vi "Spinner Facade.vi"(0 "Data In":T4, 2 "Display State In":T2, 3 "Container State":T3) -> (6 "Data Out":T4, 7 "Display State Out":T2, 8 "Action":T1)   [LabVIEW 2012, in "Spinner.xctl"]
uses:
  Spinner.xctl
  Spinner Data.ctl
  <vilib>/_xctls/Container State.ctl
  Spinner State.ctl
  <vilib>/_xctls/Action.ctl
  Command.ctl
  <vilib>/_xctls/XControlSupport.lvlib
panel:
  out "Spinner":picture
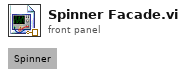
[diagram p1: front panel]
types:
  T1 = typedef "XControlSupport.lvlib/Action.ctl" = cluster{"Data Changed?":bool, "State Changed?":bool, "Action Name":string}
  T2 = typedef "Spinner.xctl/Spinner State.ctl" = cluster{"Min Speed":dbl, "Color":u32, "Max Speed":dbl, "First Run?":bool, "Value":dbl, "Refnum":refnum<vi>}
  T3 = typedef "XControlSupport.lvlib/Container State.ctl" = cluster{"Indicator?":bool, "Run Mode?":bool, " Refnum":refnum<vi>}
  T4 = typedef "Spinner.xctl/Spinner Data.ctl" = dbl
  T5 = typedef "Spinner.xctl/Command.ctl" = enum16{"Add Control", "Remove Control", "Update Imgs", "Update Speed", "Refresh"}
  T6 = typedef "LVBoundsTypeDef.ctl" = cluster{"Width":u32, "Height":u32}
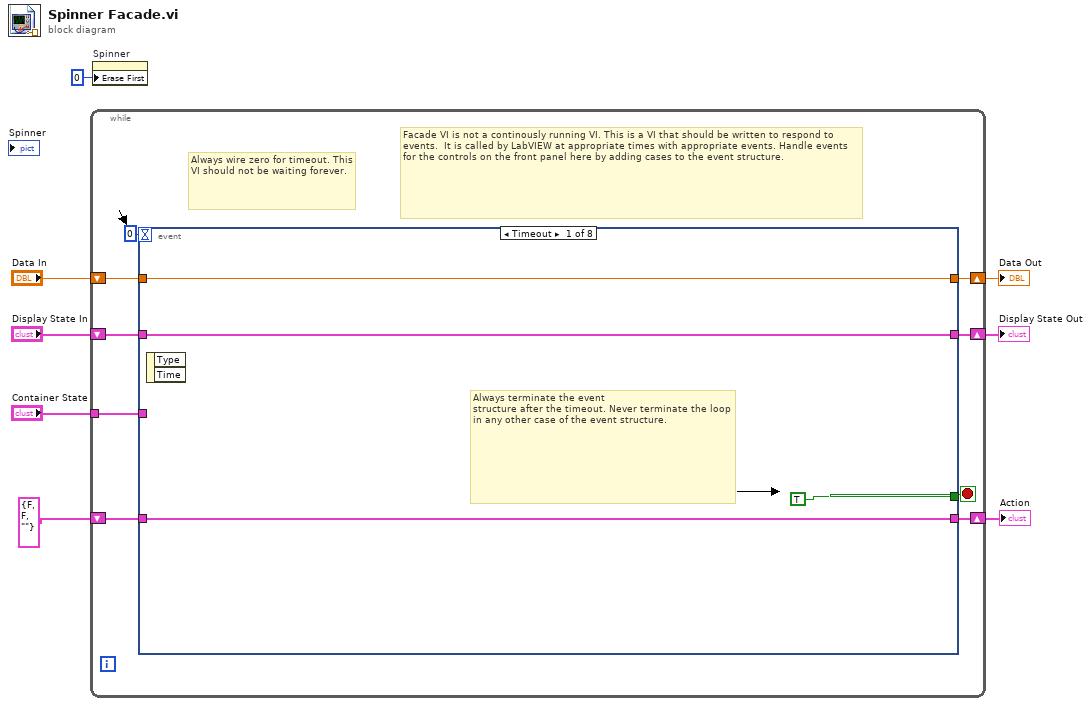
[diagram p0: block diagram]
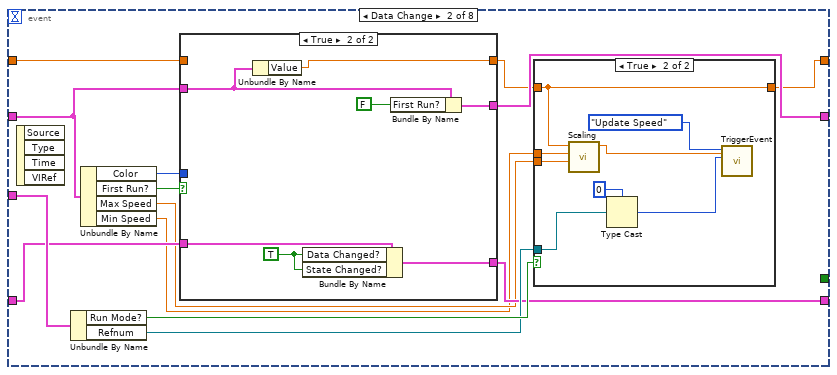
[diagram p2: hidden frame]
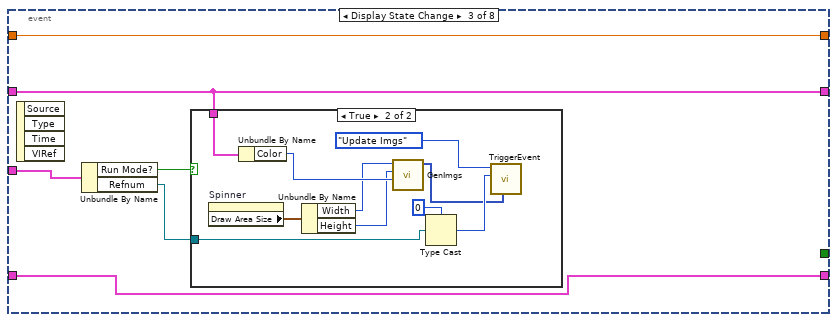
[diagram p5: hidden frame]
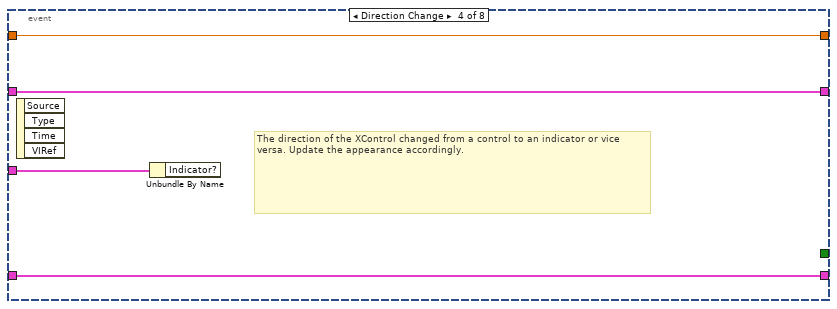
[diagram p7: hidden frame]
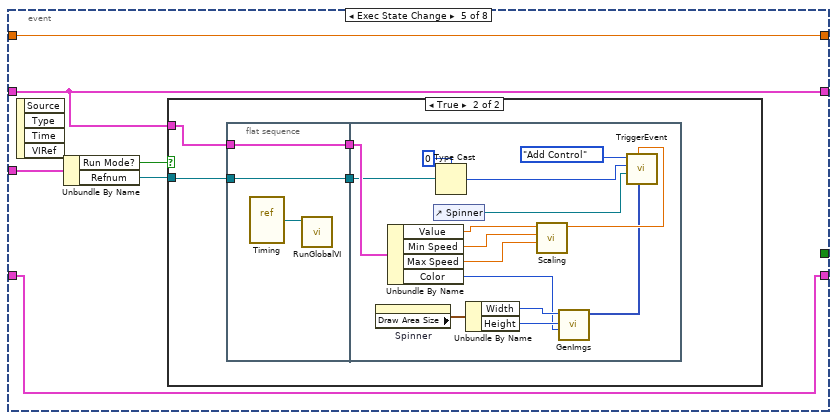
[diagram p8: hidden frame]
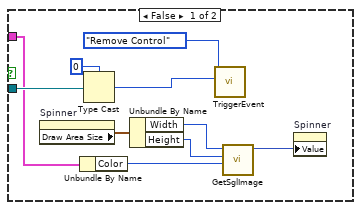
[diagram p9: hidden frame]
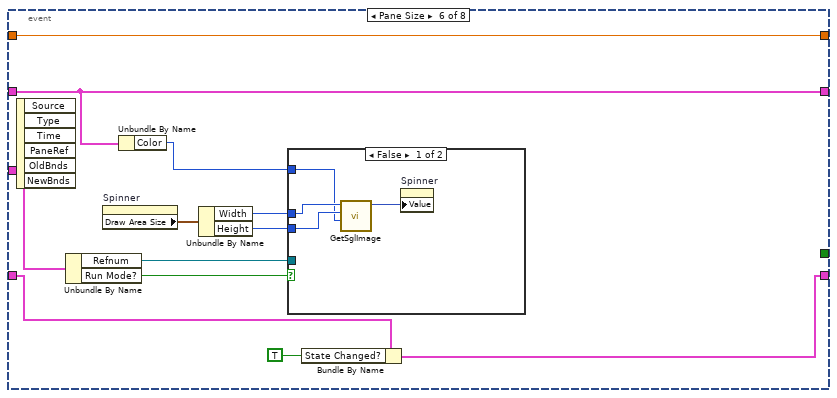
[diagram p10: hidden frame]
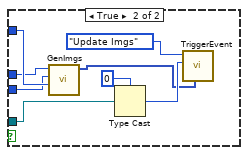
[diagram p11: hidden frame]
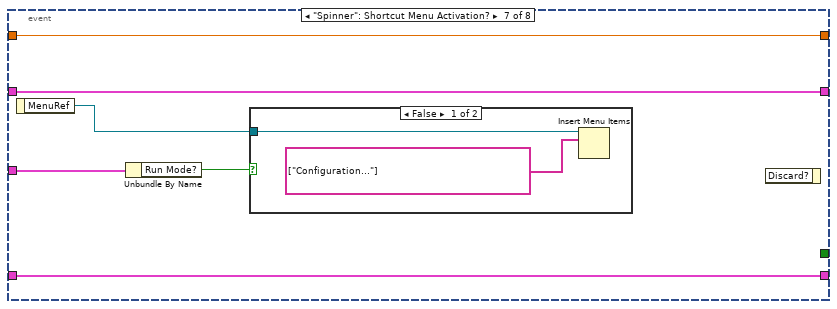
[diagram p12: hidden frame]
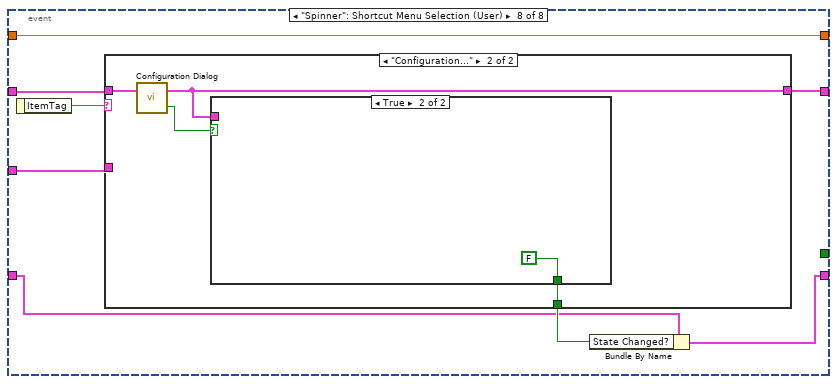
[diagram p14: hidden frame]
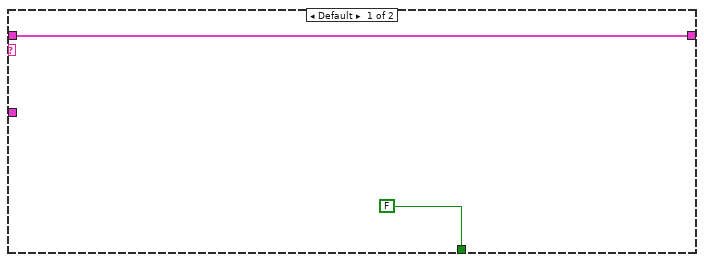
[diagram p15: hidden frame]
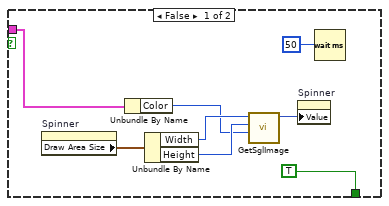
[diagram p16: hidden frame]
diagram:
  n1 = while {
    shift-right: [w16] -> w5
    shift-left: "Display State In" -> [w17]
    tunnel: "Container State" -> [w13]
    shift-right: [w11] -> w8
    shift-left: "Data In" -> [w12]
    shift-right: [w9] -> w3
    shift-left: T1 {"Data Changed?"=FALSE, "State Changed?"=FALSE, "Action Name"=""} ("Action") -> [w10]
    stop <- w15 stop-if-true
    # "Facade VI is not a continously running VI. This is a VI that should be written to respond to events.  It is called by LabVIEW at appropriate times with appropriate events. Handle events for the controls on the front panel here by adding cases to the event structure."
    # "Always wire zero for timeout. This\nVI should not be waiting forever."
    n2 = event shown="[0] Timeout" {
      selector: _ -> [_ _ _ _ _ _ _ _]
      dyn-events: _ -> [_ _ _ _ _ _ _ _]
      timeout: 0 -> [_ _ _ _ _ _ _ _]
      tunnel: w17 -> [w19 w29 w56 w73 w79 w119 w138 w148]
      tunnel: [w19 w28 w56 w73 w79 w119 w138 w145] -> w16
      tunnel: [TRUE _ _ _ _ _ _ _] -> w15
      tunnel: w13 -> [_ w35 w58 w74 w78 w124 w142 w147]
      tunnel: w12 -> [w18 w34 w59 w72 w75 w123 w139 w146]
      tunnel: [w18 w26 w59 w72 w75 w123 w139 w146] -> w11
      tunnel: [w20 w25 w60 w71 w80 w120 w137 w150] -> w9
      tunnel: w10 -> [w20 w30 w60 w71 w80 w122 w137 w151]
      event Timeout {
        # "Always terminate the event\nstructure after the timeout. Never terminate the loop in any other case of the event structure."
        n3 = event-data() -> ()  [unwired: 1 in, 2 out]
      }
      event Data Change {
        n4 = event-data() -> ()  [unwired: 1 in, 4 out]
        n5 = Unbundle By Name(w35) -> ("Run Mode?"=w33:bool, "Refnum"=w32:refnum<vi>)
        n6 = Unbundle By Name(w29) -> ("Color"=w22:u32, "First Run?"=w31:bool, "Max Speed"=w24:dbl, "Min Speed"=w23:dbl)
        n7 = case shown="True" w31 {
          tunnel: [w38 w39] -> w27
          tunnel: w34 -> [w38 _]
          tunnel: w30 -> [w36 w44]
          tunnel: w29 -> [w37 w40]
          tunnel: [w36 w42] -> w25
          tunnel: [w37 w41] -> w28
          tunnel: w22 -> [_ _]
          frame False {
          }
          frame True {
            w43 = TRUE ("Data Changed?")
            n8 = Unbundle By Name(w40) -> ("Value"=w39:dbl)
            n9 = Bundle By Name(cluster=w44, "Data Changed?"=w43, "State Changed?"=w43) -> (w42:T1)
            n10 = Bundle By Name(cluster=w40, "First Run?"=FALSE) -> (w41:T2)
          }
        }
        n11 = case shown="True" w33 {
          tunnel: w32 -> [_ w53]
          tunnel: w27 -> [w46 w52]
          tunnel: [w46 w52] -> w26
          tunnel: w24 -> [_ w51]
          tunnel: w23 -> [_ w50]
          frame False {
          }
          frame True {
            n12 = call "Scaling.vi"("max"=w51, "min"=w50, "value"=w52) -> ("Length out"=w48:dbl)  [unwired: 7 in, 1 out]
            n13 = Type Cast(type=u32 0, x=w53) -> (*(type *) &x=w49:u32)
            n14 = call "TriggerEvent.vi"("Step Len"=w48, "Ctrl Ref"=w49, "Command"=Command."Update Speed") -> ()  [unwired: 8 in, 1 out]
          }
        }
      }
      event Display State Change {
        n15 = event-data() -> ()  [unwired: 1 in, 4 out]
        n16 = Unbundle By Name(w58) -> ("Run Mode?"=w57:bool, "Refnum"=w55:refnum<vi>)
        n17 = case shown="True" w57 {
          tunnel: w56 -> [_ w67]
          tunnel: w55 -> [_ w61]
          frame False {
          }
          frame True {
            n18 = property on="Spinner" class="Pict"() -> ("Draw Area Size"=w65:T6)  [unwired: 2 in, 2 out]
            n19 = Unbundle By Name(w67) -> ("Color"=w66:u32)
            n20 = Unbundle By Name(w65) -> ("Width"=w63:u32, "Height"=w62:u32)
            n21 = call "GenImgs.vi"("Color"=w66, "Height"=w62, "Width"=w63) -> ("Imgs"=w64:picture[])  [unwired: 7 in, 1 out]
            n22 = Type Cast(type=u32 0, x=w61) -> (*(type *) &x=w69:u32)
            n23 = call "TriggerEvent.vi"("Imgs"=w64, "Ctrl Ref"=w69, "Command"=Command."Update Imgs") -> ()  [unwired: 8 in, 1 out]
          }
        }
      }
      event Direction Change {
        # "The direction of the XControl changed from a control to an indicator or vice versa. Update the appearance accordingly."
        n24 = event-data() -> ()  [unwired: 1 in, 4 out]
        n25 = Unbundle By Name(w74) -> ()  [unwired: 1 out]
      }
      event Exec State Change {
        n26 = event-data() -> ()  [unwired: 1 in, 4 out]
        n27 = Unbundle By Name(w78) -> ("Run Mode?"=w77:bool, "Refnum"=w76:refnum<vi>)
        n28 = case shown="True" w77 {
          tunnel: w79 -> [w88 w94]
          tunnel: w76 -> [w89 w93]
          frame False {
            n29 = property on="Spinner" class="Pict"() -> ("Draw Area Size"=w83:T6)  [unwired: 2 in, 2 out]
            n30 = Unbundle By Name(w88) -> ("Color"=w84:u32)
            n31 = Type Cast(type=u32 0, x=w89) -> (*(type *) &x=w87:u32)
            n32 = Unbundle By Name(w83) -> ("Width"=w82:u32, "Height"=w81:u32)
            n33 = call "TriggerEvent.vi"("Ctrl Ref"=w87, "Command"=Command."Remove Control") -> ()  [unwired: 9 in, 1 out]
            n34 = call "GetSglImage.vi"("Color"=w84, "Height"=w81, "Width"=w82) -> ("Img"=w85:picture)  [unwired: 7 in, 1 out]
            n35 = property on="Spinner" class="Pict"("Value"=w85) -> ()  [unwired: 2 in, 2 out]
          }
          frame True {
            n36 = flat-sequence {
              tunnel: w93 -> [w96]
              tunnel: w94 -> [w97]
              tunnel: [w97] -> w92
              tunnel: [w96] -> w91
              tunnel: w92 -> [w111]
              tunnel: w91 -> [w110]
              frame #0 {
                n37 = vi-ref "Timing.vi"() -> (w95:refnum<vi>)
                n38 = call "RunGlobalVI.vi"("VI input"=w95) -> ()  [unwired: 10 in, 1 out]
              }
              frame #1 {
                n39 = property on="Spinner" class="Pict"() -> ("Draw Area Size"=w103:T6)  [unwired: 2 in, 2 out]
                n40 = Unbundle By Name(w111) -> ("Value"=w98:dbl, "Min Speed"=w105:dbl, "Max Speed"=w104:dbl, "Color"=w99:u32)
                n41 = control-ref of="Spinner"() -> (w107:refnum<vi>)
                n42 = Type Cast(type=u32 0, x=w110) -> (*(type *) &x=w109:u32)
                n43 = Unbundle By Name(w103) -> ("Width"=w102:u32, "Height"=w101:u32)
                n44 = call "Scaling.vi"("max"=w104, "min"=w105, "value"=w98) -> ("Length out"=w108:dbl)  [unwired: 7 in, 1 out]
                n45 = call "GenImgs.vi"("Color"=w99, "Height"=w101, "Width"=w102) -> ("Imgs"=w100:picture[])  [unwired: 7 in, 1 out]
                n46 = call "TriggerEvent.vi"("Imgs"=w100, "Step Len"=w108, "Pic Ref"=w107, "Ctrl Ref"=w109, "Command"=Command."Add Control") -> ()  [unwired: 6 in, 1 out]
              }
            }
          }
        }
      }
      event Pane Size {
        n47 = event-data() -> ()  [unwired: 1 in, 6 out]
        n48 = Unbundle By Name(w124) -> ("Refnum"=w114:refnum<vi>, "Run Mode?"=w118:bool)
        n49 = property on="Spinner" class="Pict"() -> ("Draw Area Size"=w113:T6)  [unwired: 2 in, 2 out]
        n50 = Unbundle By Name(w119) -> ("Color"=w117:u32)
        n51 = Unbundle By Name(w113) -> ("Width"=w116:u32, "Height"=w115:u32)
        n52 = case shown="False" w118 {
          tunnel: w117 -> [w126 w134]
          tunnel: w116 -> [w128 w133]
          tunnel: w115 -> [w127 w132]
          tunnel: w114 -> [_ w129]
          frame False {
            n53 = call "GetSglImage.vi"("Color"=w126, "Height"=w127, "Width"=w128) -> ("Img"=w125:picture)  [unwired: 7 in, 1 out]
            n54 = property on="Spinner" class="Pict"("Value"=w125) -> ()  [unwired: 2 in, 2 out]
          }
          frame True {
            n55 = call "GenImgs.vi"("Color"=w134, "Height"=w132, "Width"=w133) -> ("Imgs"=w131:picture[])  [unwired: 7 in, 1 out]
            n56 = Type Cast(type=u32 0, x=w129) -> (*(type *) &x=w135:u32)
            n57 = call "TriggerEvent.vi"("Imgs"=w131, "Ctrl Ref"=w135, "Command"=Command."Update Imgs") -> ()  [unwired: 8 in, 1 out]
          }
        }
        n58 = Bundle By Name(cluster=w122, "State Changed?"=TRUE) -> (w120:T1)
      }
      event "Spinner": Shortcut Menu Activation? {
        n59 = event-data() -> ("MenuRef"=w140:refnum<k9>)  [unwired: 1 in]
        n60 = Unbundle By Name(w142) -> ("Run Mode?"=w141:bool)
        n61 = case shown="False" w141 {
          tunnel: w140 -> [w144 _]
          frame False {
            n62 = Insert Menu Items(8:string[] ["Configuration..."] ("item names"), 9:w144) -> ()  [unwired: 4 in, 3 out]
          }
          frame True {
          }
        }
        n63 = event-data() -> ()  [unwired: 2 in, 1 out]
      }
      event "Spinner": Shortcut Menu Selection (User) {
        n64 = event-data() -> ("ItemTag"=w149:string)  [unwired: 1 in]
        n65 = case shown="\"Configuration...\"" w149 {
          tunnel: w148 -> [w154 w158]
          tunnel: [w154 w155] -> w145
          tunnel: w147 -> [_ _]
          tunnel: [FALSE w156] -> w152
          frame Default {
          }
          frame "Configuration..." {
            n66 = call "Configuration Dialog.vi"("State in"=w158) -> ("Cancelled?"=w157:bool, "State out"=w155:T2)  [unwired: 1 in]
            n67 = case shown="True" w157 {
              tunnel: w155 -> [w164 _]
              tunnel: [TRUE FALSE] -> w156
              frame False {
                n68 = property on="Spinner" class="Pict"() -> ("Draw Area Size"=w163:T6)  [unwired: 2 in, 2 out]
                n69 = Unbundle By Name(w164) -> ("Color"=w160:u32)
                n70 = Unbundle By Name(w163) -> ("Width"=w162:u32, "Height"=w161:u32)
                n71 = call "GetSglImage.vi"("Color"=w160, "Height"=w161, "Width"=w162) -> ("Img"=w159:picture)  [unwired: 7 in, 1 out]
                n72 = property on="Spinner" class="Pict"("Value"=w159) -> ()  [unwired: 2 in, 2 out]
                n73 = Wait (ms)(milliseconds to wait=u32 50) -> ()  [unwired: 1 out]
              }
              frame True {
              }
            }
          }
        }
        n74 = Bundle By Name(cluster=w151, "State Changed?"=w152) -> (w150:T1)
      }
    }
  }
  "Display State Out" <- w5
  "Data Out" <- w8
  "Action" <- w3
  n75 = property on="Spinner" class="Pict"("Erase First"=u8 0) -> ()  [unwired: 2 in, 2 out]
